vi "Test Chunking.vi"() -> ()   [LabVIEW 2021]
uses:
  Typedef/Link Types.ctl
  Typedef/Format Specific/CAN Metadata.ctl
  Typedef/Format Specific/CAN Interface Mode.ctl
  Typedef/Chunk.ctl
  pcap_Parse_Build_CIF.lvclass/pcap_Parse_Build_CIF.ctl
  Build/SubVIs/Flatten SocketCAN Header.vi
  Build/Build Packet Header.vi
  Parse/Parse Packet Header.vi
  Data Accessors/Read Offset.vi
  Data Accessors/Write Offset.vi
  Utilities/Check for Global Header.vi
  Utilities/Set for Channel FIFO Format.vi
  Parse/Parse Global Header.vi
  <vilib>/CIF Foundation/CIF Utilities/DataTypes/Flatten Unflatten/Flatten U32.vi
  Build/SubVIs/Flatten Packet Header.vi
  Parse/Unflatten Packet Header.vi
  Utilities/Add Error.vi
  <vilib>/CIF Foundation/CIF Utilities/DataTypes/Flatten Unflatten/Unflatten U32.vi
  <vilib>/CIF Foundation/CIF Utilities/Errors/Append Error Location.vi
  pcap_Parse_Build_CIF.lvclass
panel:
  out "Pass":bool
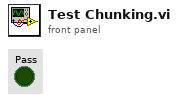
[diagram p1: front panel]
types:
  T1 = typedef "pcap_Parse_Build_CIF.lvclass/Chunk.ctl" = cluster{"Offset":i32, "Length":u32, "Start Time":i64}
  T2 = typedef "pcap_Parse_Build_CIF.lvclass/CAN Metadata.ctl" = cluster{"TAI Time (ns)":i64, "identifier":u32, "extended?":bool, "Interface Mode":T3}
  T3 = typedef "pcap_Parse_Build_CIF.lvclass/CAN Interface Mode.ctl" = enum16{"CAN 2.0", "CAN FD", "CAN FD BRS", "Remote"}
  T4 = typedef "pcap_Parse_Build_CIF.lvclass/Link Types.ctl" = enum16{"Override", "Ethernet", "Socket CAN", "I2C Linux"}
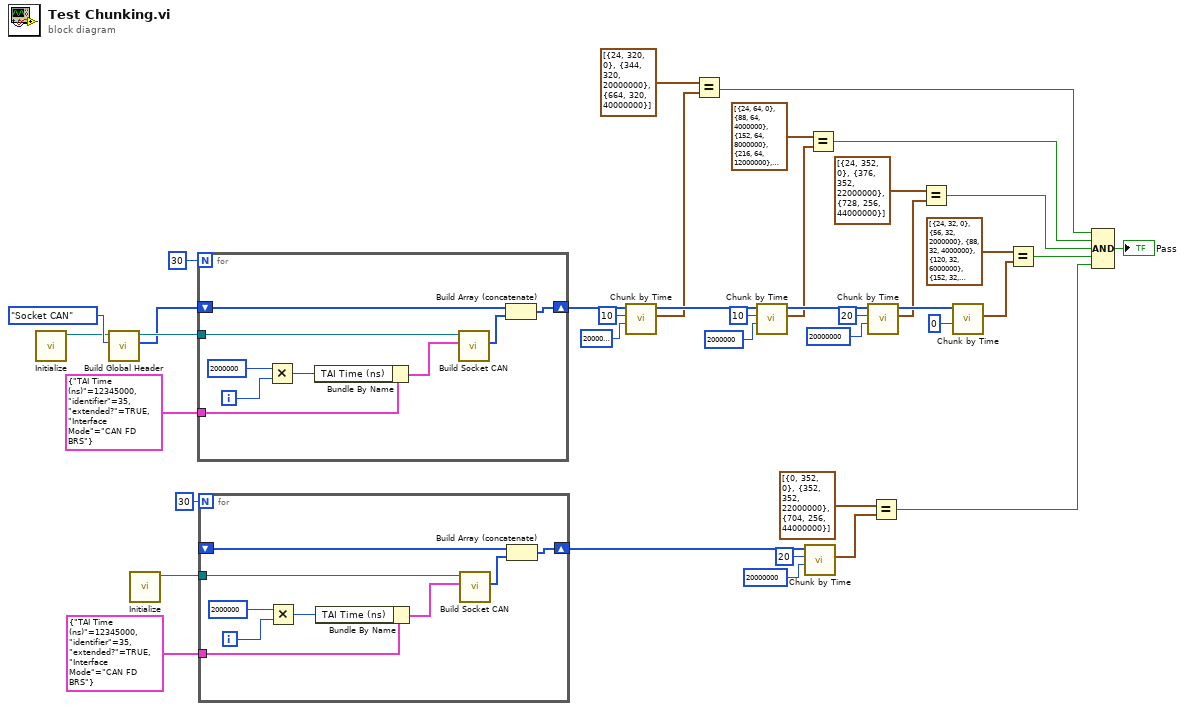
[diagram p0: block diagram]
diagram:
  n1 = call "Initialize.vi"() -> ("pcap Parse and Build out"=w37:refnum<class "pcap_Parse_Build_CIF.lvclass">)  [unwired: 11 in]
  n2 = call "Build Global Header.vi"("Link Types"=Link_Types."Socket CAN", "pcap Parse and Build in"=w37) -> ("Global Header"=w34:u8[], "pcap Parse and Build out"=w38:refnum<class "pcap_Parse_Build_CIF.lvclass">)  [unwired: 7 in, 1 out]
  n3 = call "Initialize.vi"() -> ("pcap Parse and Build out"=w13:refnum<class "pcap_Parse_Build_CIF.lvclass">)  [unwired: 11 in]
  n4 = for {
    N: 30 -> [_]
    tunnel: w38 -> [w48]
    tunnel: T2 {"TAI Time (ns)"=12345000, "identifier"=35, "extended?"=TRUE, "Interface Mode"=enum."CAN FD BRS"} ("CAN Metadata in") -> [w44]
    shift-right: [w46] -> w33
    shift-left: w34 -> [w47]
    i -> [w42]
    n5 = Multiply(x=i64 2000000, y=w42) -> (x*y=w43:i64)
    n6 = Bundle By Name(cluster=w44, "TAI Time (ns)"=w43) -> (w40:T2)
    n7 = call "Build Socket CAN.vi"("CAN Metadata"=w40, "pcap Parse and Build in"=w48) -> ("CAN Packet"=w45:u8[])  [unwired: 8 in, 1 out]
    n8 = Build Array (concatenate)(w47, w45) -> (w46:u8[])
  }
  n9 = for {
    N: 30 -> [_]
    tunnel: w13 -> [w57]
    tunnel: T2 {"TAI Time (ns)"=12345000, "identifier"=35, "extended?"=TRUE, "Interface Mode"=enum."CAN FD BRS"} ("CAN Metadata in") -> [w53]
    shift-right: [w55] -> w10
    shift-left: _ -> [w56]
    i -> [w51]
    n10 = Multiply(x=i64 2000000, y=w51) -> (x*y=w52:i64)
    n11 = Bundle By Name(cluster=w53, "TAI Time (ns)"=w52) -> (w49:T2)
    n12 = call "Build Socket CAN.vi"("CAN Metadata"=w49, "pcap Parse and Build in"=w57) -> ("CAN Packet"=w54:u8[])  [unwired: 8 in, 1 out]
    n13 = Build Array (concatenate)(w56, w54) -> (w55:u8[])
  }
  n14 = call "Chunk by Time.vi"("Time Range (ns)"=i64 200000000, "Max Frames"=10, "Bytes in"=w33) -> ("Chunks"=w22:T1[], "Bytes out"=w32:u8[])  [unwired: 7 in]
  n15 = Equal?(x=T1[] [{"Offset"=24, "Length"=320, "Start Time"=0}, {"Offset"=344, "Length"=320, "Start Time"=20000000}, {"Offset"=664, "Length"=320, "Start Time"=40000000}] ("Chunks"), y=w22) -> (x = y?=w17:bool)
  n16 = call "Chunk by Time.vi"("Time Range (ns)"=i64 2000000, "Max Frames"=10, "Bytes in"=w32) -> ("Chunks"=w4:T1[], "Bytes out"=w25:u8[])  [unwired: 7 in]
  n17 = call "Chunk by Time.vi"("Time Range (ns)"=i64 20000000, "Max Frames"=20, "Bytes in"=w10) -> ("Chunks"=w7:T1[])  [unwired: 7 in, 1 out]
  n18 = Equal?(x=T1[] [{"Offset"=24, "Length"=64, "Start Time"=0}, {"Offset"=88, "Length"=64, "Start Time"=4000000}, {"Offset"=152, "Length"=64, "Start Time"=8000000}, {"Offset"=216, "Length"=64, "Start Time"=12000000}, {"Offset"=280, "Length"=64, "Start Time"=16000000}, {"Offset"=344, "Length"=64, "Start Time"=20000000}, {"Offset"=408, "Length"=64, "Start Time"=24000000}, {"Offset"=472, "Length"=64, "Start Time"=28000000}, {"Offset"=536, "Length"=64, "Start Time"=32000000}, {"Offset"=600, "Length"=64, "Start Time"=36000000}, {"Offset"=664, "Length"=64, "Start Time"=40000000}, {"Offset"=728, "Length"=64, "Start Time"=44000000}, {"Offset"=792, "Length"=64, "Start Time"=48000000}, {"Offset"=856, "Length"=64, "Start Time"=52000000}, {"Offset"=920, "Length"=64, "Start Time"=56000000}] ("Chunks 2"), y=w4) -> (x = y?=w18:bool)
  n19 = call "Chunk by Time.vi"("Time Range (ns)"=i64 20000000, "Max Frames"=20, "Bytes in"=w25) -> ("Chunks"=w8:T1[], "Bytes out"=w24:u8[])  [unwired: 7 in]
  n20 = Equal?(x=T1[] [{"Offset"=0, "Length"=352, "Start Time"=0}, {"Offset"=352, "Length"=352, "Start Time"=22000000}, {"Offset"=704, "Length"=256, "Start Time"=44000000}] ("Chunks 5"), y=w7) -> (x = y?=w9:bool)
  n21 = Equal?(x=T1[] [{"Offset"=24, "Length"=352, "Start Time"=0}, {"Offset"=376, "Length"=352, "Start Time"=22000000}, {"Offset"=728, "Length"=256, "Start Time"=44000000}] ("Chunks 3"), y=w8) -> (x = y?=w19:bool)
  n22 = call "Chunk by Time.vi"("Time Range (ns)"=i64 0, "Bytes in"=w24) -> ("Chunks"=w21:T1[])  [unwired: 8 in, 1 out]
  n23 = Equal?(x=T1[] [{"Offset"=24, "Length"=32, "Start Time"=0}, {"Offset"=56, "Length"=32, "Start Time"=2000000}, {"Offset"=88, "Length"=32, "Start Time"=4000000}, {"Offset"=120, "Length"=32, "Start Time"=6000000}, {"Offset"=152, "Length"=32, "Start Time"=8000000}, {"Offset"=184, "Length"=32, "Start Time"=10000000}, {"Offset"=216, "Length"=32, "Start Time"=12000000}, {"Offset"=248, "Length"=32, "Start Time"=14000000}, {"Offset"=280, "Length"=32, "Start Time"=16000000}, {"Offset"=312, "Length"=32, "Start Time"=18000000}, {"Offset"=344, "Length"=32, "Start Time"=20000000}, {"Offset"=376, "Length"=32, "Start Time"=22000000}, {"Offset"=408, "Length"=32, "Start Time"=24000000}, {"Offset"=440, "Length"=32, "Start Time"=26000000}, {"Offset"=472, "Length"=32, "Start Time"=28000000}, {"Offset"=504, "Length"=32, "Start Time"=30000000}, {"Offset"=536, "Length"=32, "Start Time"=32000000}, {"Offset"=568, "Length"=32, "Start Time"=34000000}, {"Offset"=600, "Length"=32, "Start Time"=36000000}, {"Offset"=632, "Length"=32, "Start Time"=38000000}, {"Offset"=664, "Length"=32, "Start Time"=40000000}, {"Offset"=696, "Length"=32, "Start Time"=42000000}, {"Offset"=728, "Length"=32, "Start Time"=44000000}, {"Offset"=760, "Length"=32, "Start Time"=46000000}, {"Offset"=792, "Length"=32, "Start Time"=48000000}, {"Offset"=824, "Length"=32, "Start Time"=50000000}, {"Offset"=856, "Length"=32, "Start Time"=52000000}, {"Offset"=888, "Length"=32, "Start Time"=54000000}, {"Offset"=920, "Length"=32, "Start Time"=56000000}, {"Offset"=952, "Length"=32, "Start Time"=58000000}] ("Chunks 4"), y=w21) -> (x = y?=w20:bool)
  n24 = Compound Arithmetic op=AND(w17, w18, w19, w20, w9) -> (→"Pass":bool)
